vi "Check and Launch Virtual Device.vi"(7 "SCADA in":refnum<class "SCADA.lvclass">, 8 "error in (no error)":errorcluster, 11 "IED in":refnum<class "IED.lvclass">) -> (0 "error out":errorcluster, 3 "IED out":refnum<class "IED.lvclass">, 5 "SCADA out":refnum<class "SCADA.lvclass">)   [LabVIEW 2015, in "IED Actor.lvlib" / "IED.lvclass"]
uses:
  IED.lvclass
  SCADA Core/SCADA/SCADA.lvclass
  IED.lvclass/IED.ctl
  Device Specific Actors/AE75TX Actor/AE75TX/AE75TX.lvclass
  <vilib>/ActorFramework/Message Enqueuer/Message Enqueuer.lvclass
  <vilib>/ActorFramework/Actor/Actor.lvclass
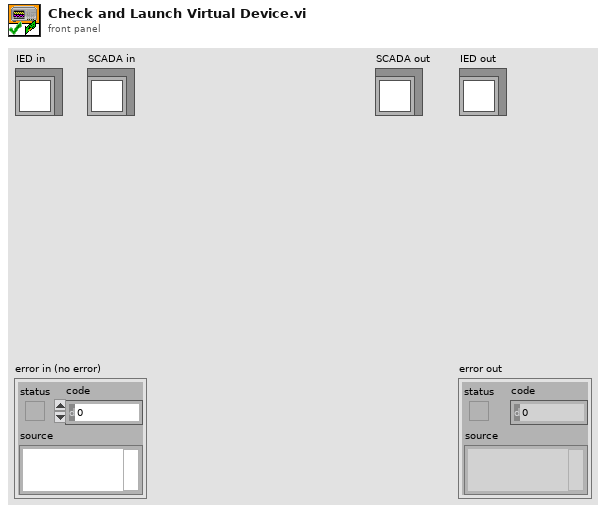
[diagram p1: front panel]
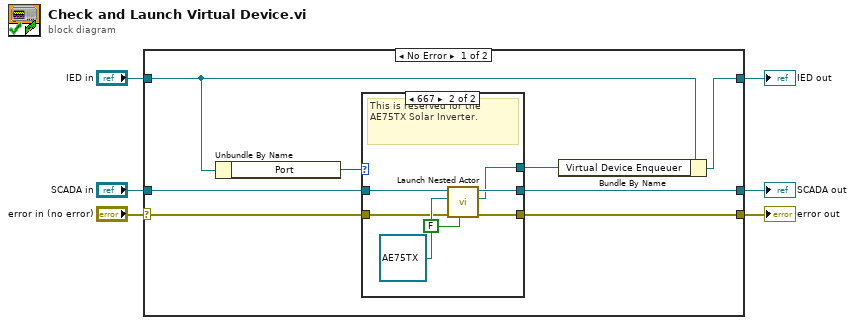
[diagram p0: block diagram]
diagram:
  n1 = case shown="No Error" "error in (no error)" {
    selector: "error in (no error)" -> [w13 w26]
    tunnel: [w11 w26] -> w5
    tunnel: [w12 w25] -> w3
    tunnel: "IED in" -> [w9 w25]
    tunnel: "SCADA in" -> [w8 w24]
    tunnel: [w7 w24] -> w1
    frame No Error {
      n2 = Unbundle By Name(w9) -> ("Port"=w14:u16)
      n3 = case shown="667" w14 {
        tunnel: w8 -> [w16 w23]
        tunnel: w13 -> [w15 w21]
        tunnel: [w16 w20] -> w7
        tunnel: [w15 w19] -> w11
        tunnel: [_ w18] -> w10
        frame 502, Default {
          # "Unless ontherwise stated, assume that the device is standard."
        }
        frame 667 {
          # "This is reserved for the AE75TX Solar Inverter."
          n4 = call <vilib>:"Launch Nested Actor.vi"("Open Actor Core front panel? (F)"=FALSE, "error in (no error)"=w21, "Nested Actor"=refnum<class "AE75TX.lvclass"> refnum ("AE75TX Actor.lvlib:AE75TX"), "Caller Actor in"=w23) -> ("error out"=w19:errorcluster, "Nested Actor's Enqueuer"=w18:refnum<class "Message Enqueuer.lvclass">, "Caller Actor out"=w20:refnum<class "SCADA.lvclass">)  [unwired: 5 in]
        }
      }
      n5 = Bundle By Name(cluster=w9, "Virtual Device Enqueuer"=w10) -> (w12:refnum<class "IED.lvclass">)
    }
    frame Error {
    }
  }
  "error out" <- w5
  "IED out" <- w3
  "SCADA out" <- w1
